vi "PythonIDE.vi"(7 "Python version":string="3.9", 9 "Processor":u16(ring) items=["SPIKE", "Pi", "Pi_ssh", "OpenMV", "duino"], 11 "Port":string) -> ()   [LabVIEW 2022 SP3]
uses:
  <vilib>/event_ctls.llb/eventvkey.ctl
  <vilib>/Utility/miscctls.llb/LVSelectionTypeDef.ctl
  06413ba0-247e-6043-8ea0-68123fbbc81b.vi
  <vilib>/Comparison/Equal/Equal Functor/Equal Functor.lvclass
  <vilib>/Platform/browser.llb/Open URL in Default Browser (string).vi
panel:
  out "live":bool
  out "last":string
  out "Text.Scroll Position":u32
  in  "Format":T1(ring)
  in  "Name":string="main.py"
  in  "Spaces":bool
  out "Shift":bool
  in  "Explorer":u16(ring) items=["Explore...", "Arm", "Backpack", "Image", "Motors", "MQTT_Client", "OnshapeTwin", "OpenMV", "Pinouts", "ROS2", "Scope", "Spatial Toolbox", "Tektronix", "Twin"]
  in  "reconnect":bool
  out "VKey":T2
  in  "Browser":bool
  out "error IO":errorcluster
  in  "Tree":string(tree)
  in  "recent":u16(ring)
  in  "CtrlE":bool
  in  "Font Size":u32=12
  in  "run":bool
  in  "Save SPIKE":bool
  out "Script":string
  in  "Python Code":string
  out "Line #":string
  out "Buffer":i32(slide) scale=0.0..100000.0
  out "History":path[](array[path])
  out "Graph":dbl[](graph)
  out "JPG":picture
  out "Chart":dbl[](graph)
  out "Console":string
  out "Path":path
  in  "Clear":bool
  in  "Ctrl C":bool
  in  "Save Log":bool
  in  "stop":bool
  # "PyVIEW IDE\nversion 0.1b37"
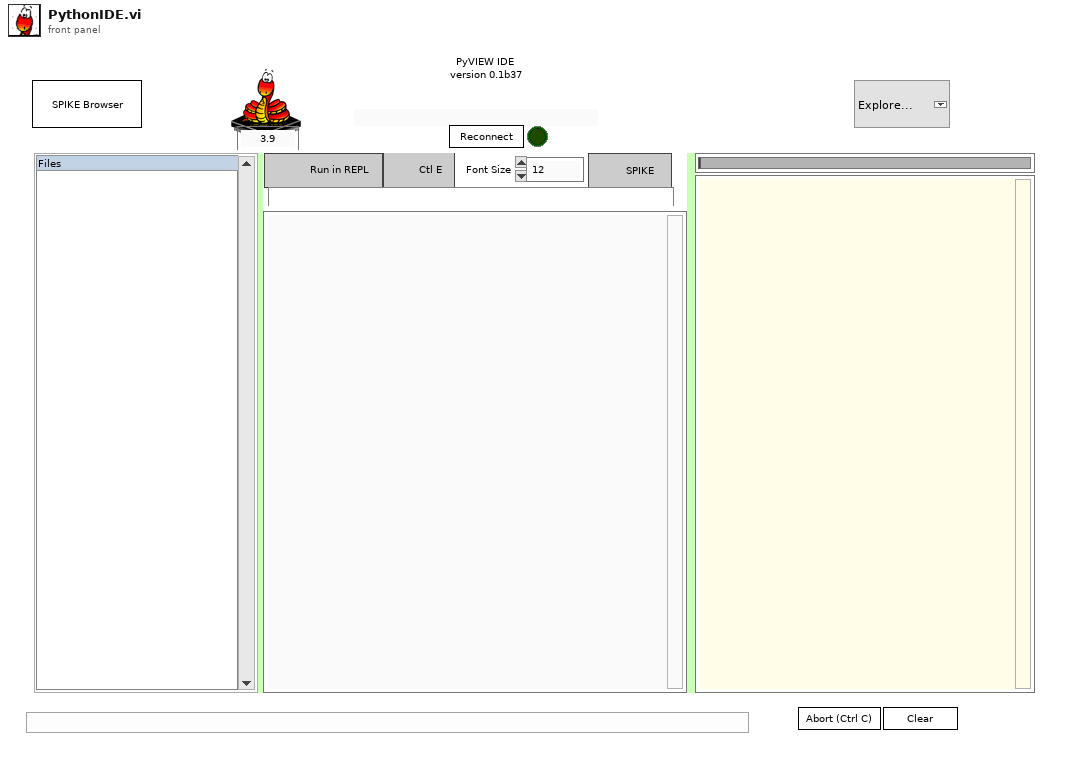
[diagram p1: front panel]
types:
  T1 = enum16{"Text", "Chart", "Waveforms", "JPEG", "Split View"}
  T2 = typedef "eventvkey.ctl" = enum16{"ASCII", "Enter", "Return", "Shift", "Ctrl", "Alt", "Cmd", "Opt", "Caps", "NumLock", "Clear", "Break", "Up", "Down", "Left", "Right", "Insert", "Delete", "Home", "End", "PageUp", "PageDown", "Escape", "Help", "Pause", "ScrollLock", "F1", "F2", "F3", "F4", "F5", "F6", "F7", "F8", "F9", "F10", "F11", "F12", "F13", "F14", "F15", "F16", "F17", "F18", "F19", "F20", "F21", "F22", "F23", "F24", "Play", "VolumeUp", "VolumeDown", "Mute", "Two Byte Char"}
  T3 = enum16{"read", "write pause", "write port", "write path", "write all"}
  T4 = typedef "PythonCtrl.ctl" = cluster{"session":refnum<k35>, "PyPath":path, "Processor":T5, "Port":string, "version":string}
  T5 = typedef "Processors.ctl" = enum16{"SPIKE", "Pi", "Pi_ssh", "OpenMV", "Dunio"}
  T6 = enum8{"Enabled", "Disabled", "Disabled and Grayed Out"}
  T7 = typedef "LVSelectionTypeDef.ctl" = cluster{"Selection Start":u32, "Selection End":u32}
  T8 = enum16{"Not data", "single values", "XY pairs", "Arrays"}
  T9 = typedef "LVPoint32TypeDef.ctl" = cluster{"Horizontal":i32, "Vertical":i32}
  T10 = typedef "Preferences.ctl" = cluster{"python":string, "arduino CLI":path, "pythonCodes":cluster{"pythonCode":path, "Color":u32}[], "FontSize":u8, "Text Colors":cluster{"Quote":u32, "function":u32, "Python":u32, "Comment":u32, "Triple Quote":u32, "Text":u32}, "SSH Logins":cluster{"IP Address":string, "Username":string, "password":string}[], "packet size":u8}
  T11 = cluster{"status":bool, "code":bool, "source":bool}
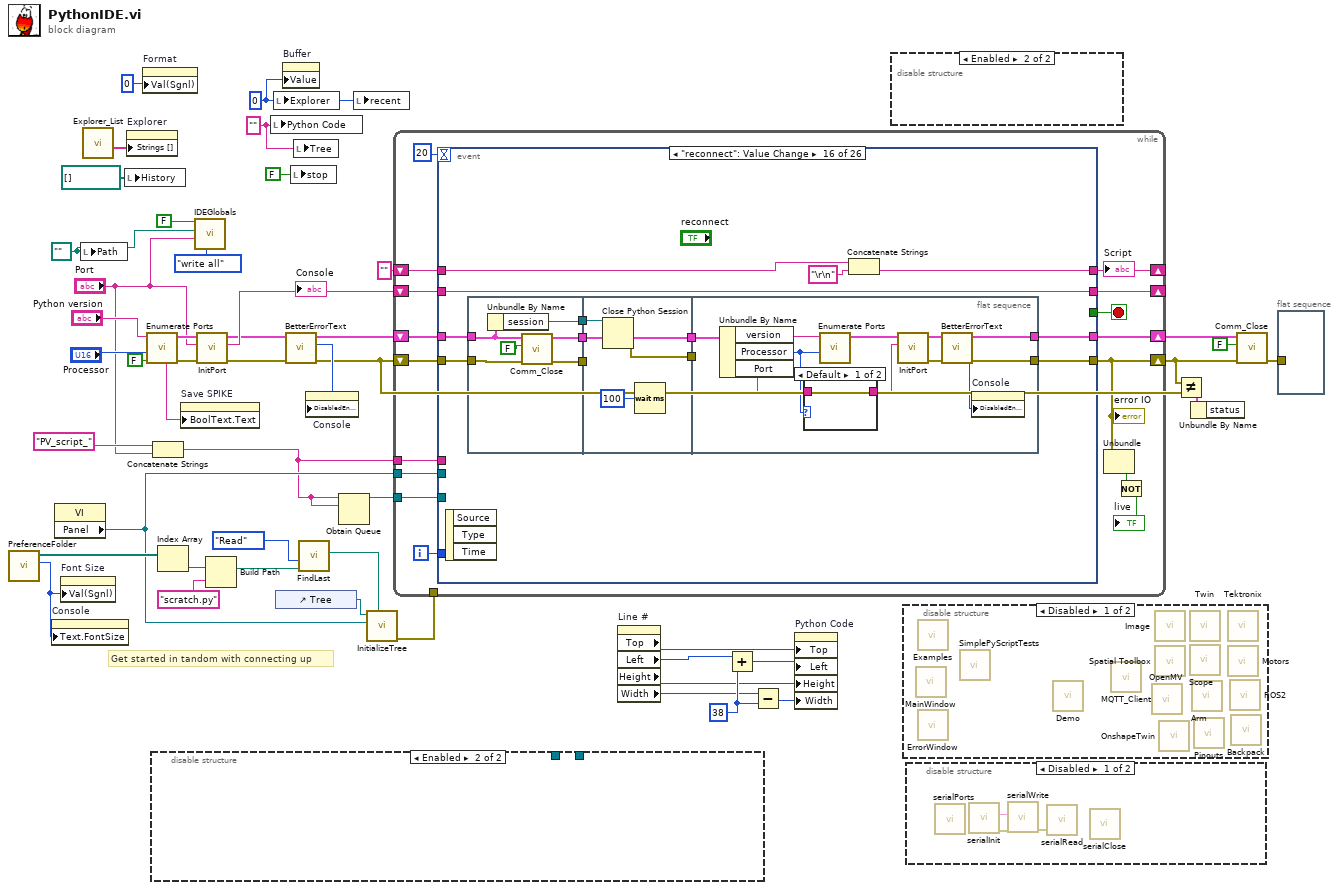
[diagram p0: block diagram]
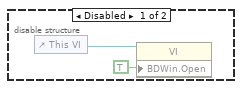
[diagram p2: hidden frame]
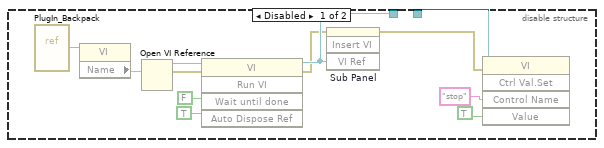
[diagram p3: hidden frame]
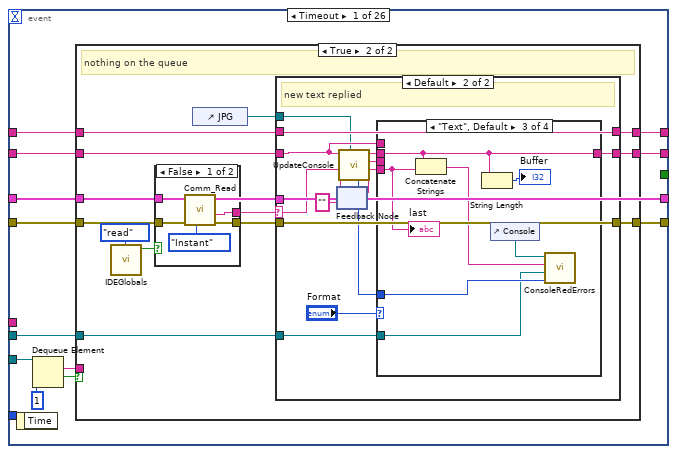
[diagram p6: hidden frame]
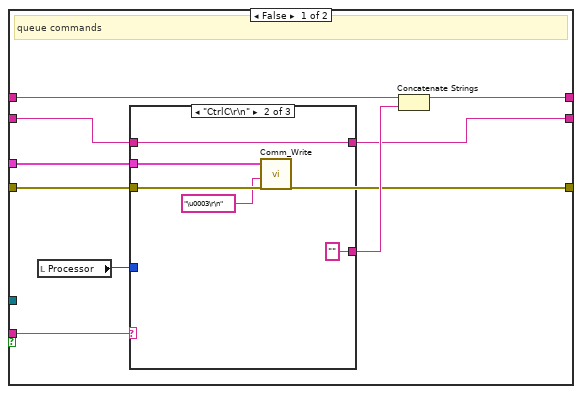
[diagram p7: hidden frame]
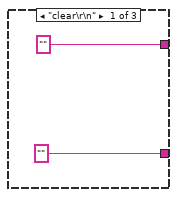
[diagram p8: hidden frame]
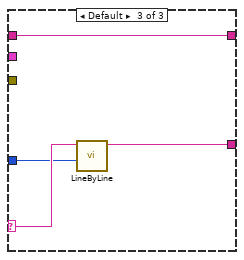
[diagram p9: hidden frame]
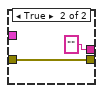
[diagram p10: hidden frame]
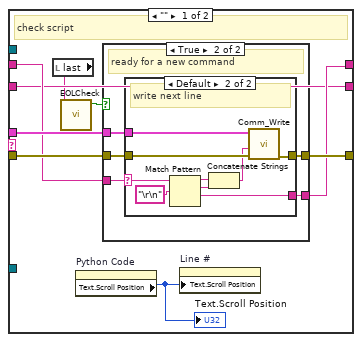
[diagram p11: hidden frame]
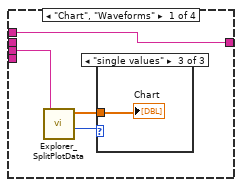
[diagram p14: hidden frame]
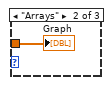
[diagram p16: hidden frame]
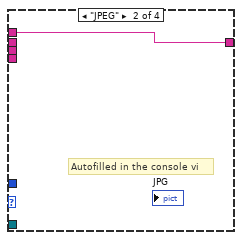
[diagram p17: hidden frame]
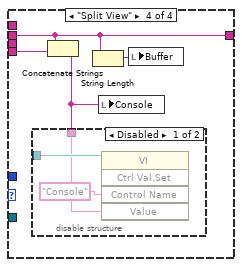
[diagram p18: hidden frame]
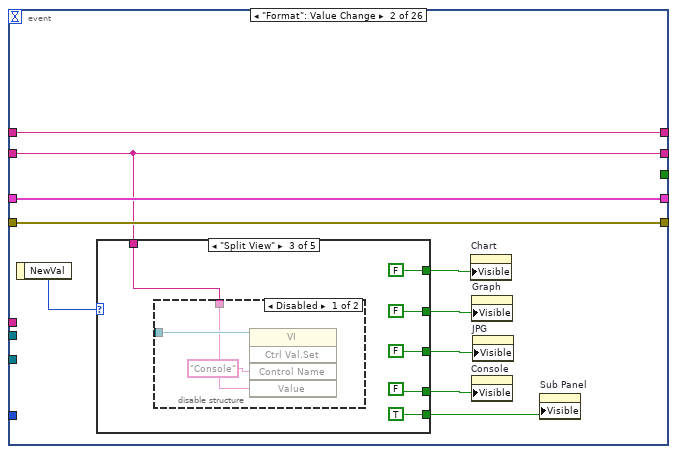
[diagram p20: hidden frame]
diagram:
  w27 = 38 ("y")
  w2 = path "" ("Path")
  w14 = 0
  w43 = "" ("Python Code")
  # "Get started in tandom with connecting up"
  n1 = call "PreferenceFolder.vi"() -> ("FontSize"=w19:u8, "pythonCodes"=w33:path[])  [unwired: 4 in, 6 out]
  n2 = property on="Console" class="Str"("Text.FontSize"=w19) -> ()  [unwired: 2 in, 2 out]
  n3 = property class="VI"() -> ("Panel"=w17:refnum<vi>)  [unwired: 2 in, 2 out]
  n4 = property on="Font Size" class="DigNum (strict)"("Val(Sgnl)"=w19) -> ()  [unwired: 2 in, 2 out]
  n5 = local write "Path"(w2) -> ()
  n6 = call "Explorer_List.vi"() -> ("Options"=w40:string[])  [unwired: 9 in, 2 out]
  n7 = local write "History"(path[] [] ("History")) -> ()
  n8 = property on="Explorer" class="Ring (strict)"("Strings []"=w40) -> ()  [unwired: 2 in, 2 out]
  n9 = property on="Format" class="Enum (strict)"("Val(Sgnl)"=0) -> ()  [unwired: 2 in, 2 out]
  n10 = call "Enumerate Ports.vi"("list?"=FALSE, "Processor"="Processor", "Python version"="Python version") -> ("error out"=w44:errorcluster, "Python"=w45:T4, "name"=w39:string)  [unwired: 3 in, 3 out]
  n11 = disable-structure shown="Enabled" {
    disable-tunnel: [w54 _] -> _
    disable-tunnel: _ -> [w51 _]
    frame Disabled {
      n12 = vi-ref "PlugIn_Backpack.vi"() -> (w55:refnum<vi>)
      n13 = property class="VI"(reference=w55) -> ("Name"=w53:string)  [unwired: 1 in, 2 out]
      n14 = Open VI Reference(vi path=w53) -> (vi reference=w57:refnum<vi>, error out=w56:errorcluster)  [unwired: 5 in]
      n15 = invoke class="VI" method="Run VI"(reference=w57, error in=w56, "Wait until done"=FALSE ("Wait Until Done"), "Auto Dispose Ref"=TRUE ("Auto Dispose Reference")) -> (reference out=w54:refnum<vi>, error out=w49:errorcluster)  [unwired: 1 in, 3 out]
      n16 = invoke on="Sub Panel" class="SubPnl" method="Insert VI"(error in=w49, "VI Ref"=w54) -> (error out=w48:errorcluster)  [unwired: 2 in, 3 out]
      n17 = invoke class="VI" method="Ctrl Val.Set"(reference=w51, error in=w48, "Control Name"="stop", "Value"=TRUE ("Auto Dispose Reference")) -> ()  [unwired: 1 in, 5 out]
    }
    frame Enabled {
    }
  }
  n18 = Concatenate Strings("PV_script_" ("name (unnamed)"), "Port") -> (w3:string)
  n19 = Index Array(array=w33) -> (element=w32:path)  [unwired: 1 in]
  n20 = property on="Save SPIKE" class="Bool"("BoolText.Text"=w39) -> ()  [unwired: 2 in, 2 out]
  n21 = call "IDEGlobals.vi"("task"=T3."write all", "Port"="Port", "Last Path"=w2, "pause?"=FALSE) -> ()  [unwired: 5 in, 3 out]
  n22 = call "InitPort.vi"("error in (no error)"=w44, "Port"="Port", "Python"=w45) -> ("error out"=w9:errorcluster, "Console"=w35:string, "Python out"=w29:T4)  [unwired: 6 in]
  "Console" <- w35
  n23 = Build Path(base path=w32, name or relative path="scratch.py" ("Python Code")) -> (appended path=w31:path)
  n24 = local write "Python Code"(w43) -> ()
  n25 = local write "Explorer"(w14) -> ()
  n26 = control-ref of="Tree"() -> (w37:refnum<vi>)
  n27 = property on="Buffer" class="Slide (strict)"("Value"=w14) -> ()  [unwired: 2 in, 2 out]
  n28 = call "BetterErrorText.vi"("error in (no error)"=w9, "Python"=w29) -> ("Disabled"=w18:T6, "Python out"=w21:T4)  [unwired: 8 in]
  n29 = local write "stop"(FALSE ("stop")) -> ()
  n30 = local write "Tree"(w43) -> ()
  n31 = call "FindLast.vi"("default"=w31, "Task"=enum16{"Save", "Read"}."Read") -> ("path"=w16:path)  [unwired: 9 in]
  n32 = property on="Console" class="Str"("DisabledEnum"=w18) -> ()  [unwired: 2 in, 2 out]
  n33 = Obtain Queue(name (unnamed)=w3, element data type=w3) -> (queue out=w41:refnum<queue>)  [unwired: 3 in, 2 out]
  n34 = local write "recent"(w14) -> ()
  n35 = call "InitializeTree.vi"("Selected File"=w16, "Panel"=w17, "TreeControl in"=w37) -> ("error out"=w11:errorcluster)  [unwired: 7 in, 1 out]
  n36 = while {
    shift-right: [w74] -> _
    shift-left: w35 -> [w75]
    shift-right: [w62] -> w10
    shift-left: w9 -> [w71]
    tunnel: w17 -> [w70]
    shift-right: [w68] -> _
    shift-left: "" -> [w69]
    tunnel: w41 -> [w66]
    shift-right: [w65] -> w13
    shift-left: w21 -> [w67]
    tunnel: w11 -> [_]
    tunnel: w3 -> [w63]
    i -> [w64]
    stop <- w73 stop-if-true
    n37 = event shown="[15] \"reconnect\": Value Change" {
      selector: _ -> [_ _ _ _ _ _ _ _ _ _ _ _ _ _ _ _ _ _ _ _ _ _ _ _ _ _]
      dyn-events: _ -> [_ _ _ _ _ _ _ _ _ _ _ _ _ _ _ _ _ _ _ _ _ _ _ _ _ _]
      timeout: 20 -> [_ _ _ _ _ _ _ _ _ _ _ _ _ _ _ _ _ _ _ _ _ _ _ _ _ _]
      tunnel: w67 -> [w77 w200 w227 w237 w253 w259 w273 w357 w366 w370 w379 w400 w417 w434 w447 w464 w496 w527 w538 w546 w553 w563 w569 w583 w592 w603]
      tunnel: w75 -> [w87 w191 w230 w244 w256 w264 w288 w360 w368 w375 w388 w398 w423 w445 w451 w465 w501 w530 w541 _ w555 w566 w578 w589 w598 w602]
      tunnel: [w86 w191 w230 w244 w256 w264 w288 w360 w368 w375 w388 w397 w423 w445 w451 w465 w501 w530 w541 w551 w555 w566 w578 w589 w598 w602] -> w74
      tunnel: [_ _ "stop" w241 _ _ _ _ _ _ _ _ _ _ _ _ _ _ _ _ _ _ _ _ _ _] -> w73
      tunnel: w71 -> [w82 w199 w229 w243 w255 w263 w282 w359 w367 w374 w387 w399 w422 w446 w452 w463 w499 w528 w539 w552 w559 w568 w580 w591 w600 w605]
      tunnel: [w85 w199 w229 w243 w255 w263 w283 w359 w367 w372 w387 w401 w422 w446 w452 w462 w499 w528 w539 w552 w559 w568 w580 w591 w600 w605] -> w62
      tunnel: w70 -> [w76 _ _ _ _ _ _ _ _ _ w386 _ _ _ _ _ _ w526 _ _ _ _ _ _ _ w608]
      tunnel: [w84 w198 w228 w242 w254 w257 w279 w361 w369 "" w385 w402 w424 w444 w450 w458 w500 w529 w540 w548 w558 w567 w579 w590 w599 w601] -> w68
      tunnel: w69 -> [w83 w198 w228 w242 w254 w262 w280 w361 w369 _ w385 w402 w424 w444 w450 w459 w500 w529 w540 w550 w558 w567 w579 w590 w599 w604]
      tunnel: w66 -> [w81 _ _ _ _ _ _ _ _ _ _ _ _ _ _ _ _ _ _ _ _ _ _ _ _ _]
      tunnel: [w77 w200 w227 w237 w253 w259 w273 w357 w366 w370 w379 w396 w417 w434 w447 w461 w496 w527 w538 w546 w553 w563 w569 w583 w592 w603] -> w65
      tunnel: w64 -> [_ _ _ _ _ _ _ _ _ _ w376 _ _ _ _ _ _ _ _ _ _ _ _ _ _ _]
      tunnel: w63 -> [_ _ _ _ _ _ _ _ _ _ _ _ w416 _ _ _ _ _ _ _ _ _ _ _ _ _]
      event Timeout {
        n38 = event-data() -> ()  [unwired: 1 in, 1 out]
        n39 = Dequeue Element(queue=w81, timeout in ms (-1)=1) -> (element=w78:string, timed out?=w79:bool)  [unwired: 1 in, 2 out]
        n40 = case shown="True" w79 {
          tunnel: w87 -> [w91 w112]
          tunnel: [w92 w114] -> w86
          tunnel: [w88 w120] -> w85
          tunnel: [w95 w119] -> w84
          tunnel: w83 -> [w96 w118]
          tunnel: w82 -> [w88 w117]
          tunnel: w77 -> [w89 w115]
          tunnel: w78 -> [w93 _]
          tunnel: w76 -> [_ w110]
          frame False {
            # "queue commands"
            n41 = local read "Processor"() -> (w90:u16)
            n42 = case shown="\"CtrlC\\r\\n\"" w93 {
              selector: w93 -> [_ _ w105]
              tunnel: ["" ("result string") "" ("result string") w107] -> w94
              tunnel: ["" ("Console") w103 w106] -> w92
              tunnel: w91 -> [_ w103 w106]
              tunnel: w90 -> [_ _ w104]
              tunnel: w89 -> [_ w100 _]
              tunnel: w88 -> [_ w99 _]
              frame "clear\r\n" {
              }
              frame "CtrlC\r\n" {
                n43 = call "Comm_Write.vi"("error in (no error)"=w99, "Text to write"="\u0003\r\n" ("function name"), "Python"=w100) -> ()  [unwired: 7 in, 2 out]
              }
              frame Default {
                n44 = call "LineByLine.vi"("Processor"=w104, "Python Code"=w105) -> ("result string"=w107:string)  [unwired: 9 in]
              }
            }
            n45 = Concatenate Strings(w96, w94) -> (w95:string)
          }
          frame True {
            # "nothing on the queue"
            n46 = call "IDEGlobals.vi"("task"=T3."read") -> ("pause? out"=w108:bool)  [unwired: 8 in, 2 out]
            n47 = case shown="False" w108 {
              tunnel: w117 -> [w125 w127]
              tunnel: [w124 "" ("Text read")] -> w113
              tunnel: [w123 w127] -> w116
              tunnel: w115 -> [w122 _]
              frame False {
                n48 = call "Comm_Read.vi"("Task"=enum16{"Instant", "All"}."Instant", "error in (no error)"=w125, "Python"=w122) -> ("error out"=w123:errorcluster, "Text read"=w124:string)  [unwired: 7 in]
              }
              frame True {
              }
            }
            n49 = control-ref of="JPG"() -> (w111:refnum<vi>)
            n50 = case shown="Default" w113 {
              selector: w113 -> [_ w162]
              tunnel: w112 -> [w130 w157]
              tunnel: w116 -> [w136 w169]
              tunnel: [w135 w169] -> w120
              tunnel: w118 -> [w133 w168]
              tunnel: [w132 w168] -> w119
              tunnel: w115 -> [w134 _]
              tunnel: [w130 w158] -> w114
              tunnel: w111 -> [_ w156]
              tunnel: w110 -> [_ w155]
              frame "" {
                # "check script"
                n51 = local read "last"() -> (w128:string)
                n52 = call "EOLCheck.vi"("Console"=w128) -> ("waiting...."=w129:bool)  [unwired: 10 in]
                n53 = property on="Python Code" class="Str"() -> ("Text.Scroll Position"=w131:u32)  [unwired: 2 in, 2 out]
                "Text.Scroll Position" <- w131
                n54 = case shown="True" w129 {
                  tunnel: w136 -> [w138 w143]
                  tunnel: [w138 w142] -> w135
                  tunnel: w134 -> [_ w141]
                  tunnel: w133 -> [w137 w140]
                  tunnel: [w137 w139] -> w132
                  frame False {
                  }
                  frame True {
                    # "ready for a new command"
                    n55 = case shown="Default" w140 {
                      selector: w140 -> [w144 w146]
                      tunnel: [w144 w154] -> w139
                      tunnel: w143 -> [w145 w150]
                      tunnel: [w145 w149] -> w142
                      tunnel: w141 -> [_ w147]
                      frame "" {
                      }
                      frame Default {
                        # "write next line"
                        n56 = Match Pattern(string=w146, regular expression="\r\n") -> (before substring=w152:string, match substring=w151:string, after substring=w154:string)  [unwired: 1 in, 1 out]
                        n57 = Concatenate Strings(w152, w151) -> (w148:string)
                        n58 = call "Comm_Write.vi"("error in (no error)"=w150, "Text to write"=w148, "Python"=w147) -> ("error out"=w149:errorcluster)  [unwired: 7 in, 1 out]
                      }
                    }
                  }
                }
                n59 = property on="Line #" class="Str"("Text.Scroll Position"=w131) -> ()  [unwired: 2 in, 2 out]
              }
              frame Default {
                # "new text replied"
                n60 = feedback #1("" ("Left over raw")) -> (w166:string)
                n61 = call "UpdateConsole.vi"("JPG"=w156, "from last time raw"=w166, "New Text"=w162, "Console"=w157) -> ("Left over raw"=w167:string, "left over fixed"=w160:string, "LastFullLine"=w161:string, "Console Out"=w159:string, "cursor out"=w164:i32)  [unwired: 2 in, 1 out]
                n62 = feedback-in #1(w167) -> ()
                n63 = case shown="\"Text\", Default" "Format" {
                  tunnel: w164 -> [_ _ w183 _]
                  tunnel: w161 -> [w173 _ _ _]
                  tunnel: w159 -> [_ _ w180 w186]
                  tunnel: w160 -> [_ _ w181 w187]
                  tunnel: [w170 w176 w180 w186] -> w158
                  tunnel: w157 -> [w170 w176 _ _]
                  tunnel: w155 -> [_ _ w178 _]
                  frame "Chart", "Waveforms" {
                    n64 = call "Explorer_SplitPlotData.vi"("Value"=w173) -> ("Data type"=w171:T8, "Array"=w172:dbl[])  [unwired: 9 in]
                    n65 = case shown="\"single values\"" w171 {
                      tunnel: w172 -> [_ w174 w175]
                      frame Default {
                      }
                      frame "Arrays" {
                        "Graph" <- w174
                      }
                      frame "single values" {
                        "Chart" <- w175
                      }
                    }
                  }
                  frame "JPEG" {
                    # "Autofilled in the console vi"
                  }
                  frame "Text", Default {
                    n66 = Concatenate Strings(w180, w181) -> (w177:string)
                    n67 = String Length(string=w180) -> (length=→"Buffer":i32)
                    n68 = control-ref of="Console"() -> (w179:refnum<vi>)
                    n69 = call "ConsoleRedErrors.vi"("Text.Selection:End"=w183, "Front Panel"=w178, "Console in"=w177, "String in"=w179) -> ()  [unwired: 6 in, 2 out]
                    "last" <- w181
                  }
                  frame "Split View" {
                    n70 = Concatenate Strings(w186, w187) -> (w184:string)
                    n71 = disable-structure shown="Disabled" {
                      disable-tunnel: _ -> [w189 _]
                      disable-tunnel: w184 -> [w188 _]
                      frame Disabled {
                        n72 = invoke class="VI" method="Ctrl Val.Set"(reference=w189, "Control Name"="Console", "Value"=w188) -> ()  [unwired: 2 in, 5 out]
                      }
                      frame Enabled {
                      }
                    }
                    n73 = String Length(string=w186) -> (length=w185:i32)
                    n74 = local write "Console"(w184) -> ()
                    n75 = local write "Buffer"(w185) -> ()
                  }
                }
              }
            }
          }
        }
      }
      event "Format": Value Change {
        n76 = event-data() -> ("NewVal"=w197:T1)  [unwired: 1 in]
        n77 = case shown="\"Split View\"" w197 {
          tunnel: [TRUE ("Visible") FALSE ("Visible") FALSE ("Visible") FALSE ("Visible") FALSE ("Visible")] -> w196
          tunnel: [FALSE ("Visible") TRUE ("Visible") FALSE ("Visible") FALSE ("Visible") FALSE ("Visible")] -> w195
          tunnel: [FALSE ("Visible") FALSE ("Visible") FALSE ("Visible") TRUE ("Visible") FALSE ("Visible")] -> w194
          tunnel: [FALSE ("Visible") FALSE ("Visible") FALSE ("Visible") FALSE ("Visible") TRUE ("Visible")] -> w193
          tunnel: [_ FALSE ("Visible") TRUE ("Visible") _ _] -> w192
          tunnel: w191 -> [_ _ w210 _ _]
          frame "JPEG" {
          }
          frame "Waveforms" {
          }
          frame "Split View" {
            n78 = disable-structure shown="Disabled" {
              disable-tunnel: _ -> [w217 _]
              disable-tunnel: w210 -> [w216 _]
              frame Disabled {
                n79 = invoke class="VI" method="Ctrl Val.Set"(reference=w217, "Control Name"="Console", "Value"=w216) -> ()  [unwired: 2 in, 5 out]
              }
              frame Enabled {
              }
            }
          }
          frame "Chart" {
          }
          frame "Text" {
          }
        }
        n80 = property on="Chart" class="WFChart (strict)"("Visible"=w194) -> ()  [unwired: 2 in, 2 out]
        n81 = property on="Graph" class="WFGraph (strict)"("Visible"=w195) -> ()  [unwired: 2 in, 2 out]
        n82 = property on="Console" class="Str"("Visible"=w193) -> ()  [unwired: 2 in, 2 out]
        n83 = property on="JPG" class="Pict"("Visible"=w196) -> ()  [unwired: 2 in, 2 out]
        n84 = property on="Sub Panel" class="SubPnl"("Visible"=w192) -> ()  [unwired: 2 in, 2 out]
      }
      event "stop": Value Change {
        n85 = event-data() -> ()  [unwired: 1 in, 1 out]
      }
      event Panel Close? {
        w236 = "" ("source")
        w241 = TRUE ("stop")
        n86 = event-data() -> ()  [unwired: 1 in, 3 out]
        n87 = control-ref of="Tree"() -> (w240:refnum<vi>)
        n88 = property on="recent" class="Ring (strict)"("Strings []"=string[] []) -> ()  [unwired: 2 in, 2 out]
        n89 = invoke on="Invoke Node" class="Tree (strict)" method="Edit Tree Items.Delete"(reference=w240, "Delete Children"=TRUE ("Delete Children?")) -> ()  [unwired: 3 in, 5 out]
        n90 = local write "Python Code"(w236) -> ()
        n91 = local write "Console"(w236) -> ()
        n92 = local write "Path"(path "") -> ()
        n93 = local write "Line #"(w236) -> ()
        n94 = local write "History"(path[] [] ("History")) -> ()
        n95 = property on="Console" class="Str"("Visible"=TRUE ("Delete Children?")) -> ()  [unwired: 2 in, 2 out]
        n96 = property on="Sub Panel" class="SubPnl"("Visible"=FALSE ("Delete Children?")) -> ()  [unwired: 2 in, 2 out]
        n97 = event-data("Discard?"=w241) -> ()  [unwired: 1 in, 1 out]
      }
      event Pane Size; Panel Resize {
        w247 = 38 ("y")
        n98 = event-data() -> ()  [unwired: 1 in, 5 out]
        n99 = property on="Line #" class="Str"() -> ("Top"=w250:i32, "Left"=w252:i32, "Height"=w249:u32, "Width"=w248:u32)  [unwired: 2 in, 2 out]
        n100 = local read "Text.Scroll Position"() -> (w245:u32)
        n101 = Add(x=w252, y=w247) -> (x+y=w251:i32)
        n102 = Subtract(x=w248, y=w247) -> (x-y=w246:u32)
        n103 = property on="Python Code" class="Str"("Text.Scroll Position"=w245, "Top"=w250, "Left"=w251, "Height"=w249, "Width"=w246) -> ()  [unwired: 2 in, 2 out]
      }
      event "run": Value Change {
        n104 = event-data() -> ()  [unwired: 1 in, 1 out]
        n105 = local read "Processor"() -> (w260:u16)
        n106 = case shown="False" "CtrlE" {
          tunnel: [w267 w270] -> w257
          tunnel: "Python Code" -> [w266 w271]
          tunnel: w260 -> [w265 _]
          frame False {
            n107 = call "LineByLine.vi"("Processor"=w265, "Python Code"=w266) -> ("result string"=w267:string)  [unwired: 9 in]
          }
          frame True {
            n108 = Concatenate Strings("\u0005" ("string"), w271, "\u0004" ("string")) -> (w270:string)
          }
        }
        n109 = Concatenate Strings(w262, w257) -> ()  [unwired: 1 out]
      }
      event Key Down? {
        n110 = event-data() -> ("PlatMods.Shift"=w274:bool, "PlatMods.Cmd"=w284:bool, "PlatMods.Ctrl"=w285:bool, "Char"=w286:i16, "VKey"=w287:T2)  [unwired: 1 in]
        "VKey" <- w287
        "Shift" <- w274
        n111 = property on="Python Code" class="Str"() -> ("Key Focus"=w276:bool)  [unwired: 2 in, 2 out]
        n112 = property on="Sub Panel" class="SubPnl"() -> ("Key Focus"=w272:bool)  [unwired: 2 in, 2 out]
        n113 = property on="Name" class="Str"() -> ("Key Focus"=w277:bool)  [unwired: 2 in, 2 out]
        n114 = Compound Arithmetic op=OR(w272, w276, w277) -> (w275:bool)
        n115 = case shown="True" w275 {
          tunnel: w273 -> [w297 _]
          tunnel: w287 -> [w299 _]
          tunnel: w286 -> [w298 w350]
          tunnel: w285 -> [w290 _]
          tunnel: w284 -> [w291 _]
          tunnel: [w295 w352] -> w283
          tunnel: w282 -> [w296 w352]
          tunnel: [w292 w349] -> w281
          tunnel: w280 -> [w294 w351]
          tunnel: [w293 w351] -> w279
          tunnel: w274 -> [_ w348]
          frame False {
            n116 = Or(x=w291, y=w290) -> (x .or. y?=w289:bool)
            n117 = case shown="True" w289 {
              tunnel: w299 -> [w306 _]
              tunnel: w298 -> [w305 w322]
              tunnel: w297 -> [w304 w321]
              tunnel: w296 -> [w303 w320]
              tunnel: [w301 w319] -> w295
              tunnel: w294 -> [w300 w318]
              tunnel: [w300 w317] -> w293
              tunnel: w291 -> [_ w316]
              tunnel: [_ w315] -> w292
              frame False {
                n118 = case shown="\"Left\"" w306 {
                  tunnel: w305 -> [_ _ _ _ _ w314]
                  tunnel: ["\r\n" ("replace string (\"\")") "\u001b[A" ("replace string (\"\")") "\u001b[B" ("replace string (\"\")") "\u001b[D" ("replace string (\"\")") "\u001b[C" ("replace string (\"\")") w312] -> w302
                  frame "Enter", "Return" {
                  }
                  frame "Up" {
                  }
                  frame "Down" {
                  }
                  frame "Left" {
                  }
                  frame "Right" {
                  }
                  frame Default {
                    n119 = Build Array(w314) -> (w313:i16[])
                    n120 = Byte Array To String(unsigned byte array=w313) -> (string=w312:string)
                  }
                }
                n121 = call "Comm_Write.vi"("error in (no error)"=w303, "Text to write"=w302, "Python"=w304) -> ("error out"=w301:errorcluster)  [unwired: 7 in, 1 out]
              }
              frame True {
                n122 = case shown="Default" w322 {
                  selector: w322 -> [w325 _]
                  tunnel: w321 -> [w330 _]
                  tunnel: w320 -> [w329 w347]
                  tunnel: [w328 w347] -> w319
                  tunnel: w318 -> [w326 w346]
                  tunnel: [w326 w345] -> w317
                  tunnel: w316 -> [w324 _]
                  tunnel: [w323 _] -> w315
                  frame Default {
                    n123 = case shown="False" w324 {
                      tunnel: [w332 "" ("string")] -> w327
                      tunnel: w325 -> [w331 _]
                      tunnel: [_ TRUE ("Discard?")] -> w323
                      frame False {
                        # "Ctrl - clean up"
                        n124 = case shown="98" w331 {
                          tunnel: w331 -> [_ _ _ _ w338]
                          tunnel: ["\u0003" ("string") "\u0002" ("string") "\u0004" ("string") "\u0005" ("string") w337] -> w332
                          frame 67, 99 {
                          }
                          frame 98 {
                            # "Ctrl B PC"
                          }
                          frame 68, 100 {
                          }
                          frame 101 {
                            # "Ctrl E PC"
                          }
                          frame Default {
                            # "Ctrl C PC"
                            n125 = Build Array(w338) -> (w339:i16[])
                            n126 = Byte Array To String(unsigned byte array=w339) -> (string=w337:string)
                          }
                        }
                      }
                      frame True {
                        # "Cmd C/V use OS"
                      }
                    }
                    n127 = call "Comm_Write.vi"("error in (no error)"=w329, "Text to write"=w327, "Python"=w330) -> ("error out"=w328:errorcluster)  [unwired: 7 in, 1 out]
                  }
                  frame 22, 118 {
                    # "paste"
                    n128 = invoke class="App" method="Clipboard.Read"() -> ("Read Clipbrd"=w344:string)  [unwired: 3 in, 2 out]
                    n129 = local read "Processor"() -> (w342:u16)
                    n130 = call "LineByLine.vi"("Processor"=w342, "Python Code"=w344) -> ("result string"=w343:string)  [unwired: 9 in]
                    n131 = Concatenate Strings(w346, w343) -> (w345:string)
                  }
                }
              }
            }
          }
          frame True {
            n132 = case shown="9" w350 {
              tunnel: [TRUE ("Discard?") _] -> w349
              tunnel: w348 -> [_ w355]
              frame 0, Default {
              }
              frame 9 {
                # "Tab key"
                n133 = control-ref of="Python Code"() -> (w356:refnum<vi>)
                n134 = call "Tab_In_Out.vi"("Shift?"=w355, "String in"=w356) -> ("result string"=w354:string)  [unwired: 9 in]
                n135 = property on="Python Code" class="Str"("Val(Sgnl)"=w354) -> ()  [unwired: 2 in, 2 out]
              }
            }
          }
        }
        n136 = Not(x=w281) -> (.not. x?=w278:bool)
        n137 = event-data("Discard?"=w278) -> ()  [unwired: 1 in, 1 out]
      }
      event Key Up {
        n138 = event-data() -> ()  [unwired: 1 in, 8 out]
        n139 = local write "Shift"(FALSE ("Shift")) -> ()
      }
      event "recent": Value Change {
        n140 = event-data() -> ()  [unwired: 1 in, 6 out]
        n141 = local read "History"() -> (w364:path[])
        n142 = Index Array(array=w364, index="recent") -> (element=w363:path)
        n143 = Path To String(path=w363) -> (string=w362:string)
        n144 = property on="Tree" class="Tree (strict)"("Val(Sgnl)"=w362) -> ()  [unwired: 2 in, 2 out]
      }
      event "Ctrl C": Value Change {
        n145 = event-data() -> ()  [unwired: 1 in, 1 out]
        n146 = call "Comm_Write.vi"("error in (no error)"=w374, "Text to write"="\u0003\r\n\r\n" ("function name"), "Python"=w370) -> ("error out"=w372:errorcluster)  [unwired: 7 in, 1 out]
      }
      event "Python Code": Value Change {
        n147 = event-data() -> ()  [unwired: 1 in, 1 out]
        n148 = local read "VKey"() -> (w383:T2)
        n149 = case shown="\"Enter\", \"Return\"" w383 {
          tunnel: [FALSE TRUE] -> w382
          frame Default {
          }
          frame "Enter", "Return" {
          }
        }
        n150 = control-ref of="Python Code"() -> (w384:refnum<vi>)
        n151 = call "Color_Assign.vi"("Add Spaces?"=w382, "Front Panel"=w386, "Code"=w384) -> ("Value"=w378:string)  [unwired: 8 in]
        n152 = call "BuildLineNumbers.vi"("Python Code"=w378) -> ("String"=→"Line #":string)  [unwired: 10 in]
        n153 = property on="Python Code" class="Str"() -> ("DisabledEnum"=w380:T6)  [unwired: 2 in, 2 out]
        n154 = local read "Tree"() -> (w381:string)
        n155 = case shown="\"Enabled\"" w380 {
          tunnel: w378 -> [_ w392]
          tunnel: w381 -> [_ w391]
          tunnel: w376 -> [_ w389]
          frame Default {
          }
          frame "Enabled" {
            n156 = case shown="0..5" w389 {
              frame Default {
              }
              frame 0..5 {
                n157 = property on="Ctrl C" class="Bool"("Key Focus"=TRUE) -> ()  [unwired: 2 in, 2 out]
              }
            }
            n158 = String To Path(string=w391) -> (path=w390:path)
            n159 = Write to Text File(file (use dialog)=w390, text=w392) -> ()  [unwired: 2 in, 3 out]
          }
        }
      }
      event "Save SPIKE": Value Change {
        n160 = event-data() -> ()  [unwired: 1 in, 3 out]
        n161 = case shown="No Error" w399 {
          selector: w399 -> [w410 w415]
          tunnel: [w412 w415] -> w401
          tunnel: w398 -> [_ w414]
          tunnel: w400 -> [w411 w413]
          tunnel: [w404 w414] -> w397
          tunnel: [w403 w413] -> w396
          frame No Error {
            n162 = local read "Tree"() -> (w407:string)
            n163 = local read "Python Code"() -> (w409:string)
            n164 = String To Path(string=w407) -> (path=w408:path)
            n165 = Strip Path(path=w408) -> (name=w406:string)  [unwired: 1 out]
            n166 = control-ref of="Console"() -> (w405:refnum<vi>)
            n167 = call "UploadFiles.vi"("Code"=w409, "error in (no error)"=w410, "Python in"=w411, "name"=w406, "Console"=w405) -> ("error out"=w412:errorcluster, "Console out"=w404:string, "Python out"=w403:T4)  [unwired: 4 in]
          }
          frame Error {
          }
        }
      }
      event "Explorer": Value Change {
        n168 = event-data() -> ("NewVal"=w419:u16)  [unwired: 1 in]
        n169 = property on="Explorer" class="Ring (strict)"() -> ("Strings []"=w420:string[])  [unwired: 2 in, 2 out]
        n170 = Index Array(array=w420, index=w419) -> (element=w418:string)
        n171 = case shown="Default" w419 {
          tunnel: w418 -> [_ w431]
          tunnel: w416 -> [_ w425]
          frame 0 {
          }
          frame Default {
            n172 = local read "Shift"() -> (w430:bool)
            n173 = Select(t=enum16{"run", "open"}."open" ("Task"), s=w430, f=enum16{"run", "open"}."run" ("Task")) -> (s? t:f=w427:enum16{"run", "open"})
            n174 = control-ref of="Console"() -> (w432:refnum<vi>)
            n175 = control-ref of="JPG"() -> (w426:refnum<vi>)
            n176 = call "Explore_Open.vi"("JPG"=w426, "Task"=w427, "queueName"=w425, "Name"=w431, "String in"=w432) -> ()  [unwired: 7 in]
          }
        }
        n177 = local write "Explorer"(0) -> ()
      }
      event "Browser": Value Change {
        w442 = 128  # call and forget
        n178 = event-data() -> ()  [unwired: 1 in, 3 out]
        n179 = vi-ref "Examples.vi"() -> (w439:refnum<vi>)
        n180 = property class="VI"(reference=w439) -> ("Name"=w440:string)  [unwired: 1 in, 2 out]
        n181 = local read "Python version"() -> (w433:string)
        n182 = local read "Port"() -> (w438:string)
        n183 = Open VI Reference(type specifier VI Refnum (for type only)=refnum<vi> refnum, vi path=w440, options=w442) -> (vi reference=w443:refnum<vi>, error out=w435:errorcluster)  [unwired: 3 in]
        n184 = call-by-ref "Start Asynchronous Call"(reference=w443, error in=w435, "Python version"=w433, "Python"=w434, "Port"=w438) -> (reference out=w436:refnum<vi>, error out=w437:errorcluster)  [unwired: 9 in]
        n185 = Close Reference(reference=w436, error in (no error)=w437) -> ()  [unwired: 1 out]
      }
      event "Spaces": Value Change {
        n186 = event-data() -> ()  [unwired: 1 in, 3 out]
        n187 = property on="Python Code" class="Str"() -> ("Value"=w448:string)  [unwired: 2 in, 2 out]
        n188 = call "CleanUp.vi"("Python Code"=w448) -> ("spreadsheet string"=w449:string)  [unwired: 10 in]
        n189 = property on="Python Code" class="Str"("Val(Sgnl)"=w449) -> ()  [unwired: 2 in, 2 out]
      }
      event "reconnect": Value Change {
        n190 = event-data() -> ()  [unwired: 1 in, 3 out]
        n191 = flat-sequence {
          tunnel: w464 -> [w468]
          tunnel: w463 -> [w470]
          tunnel: [w469] -> w457
          tunnel: [w468] -> w455
          tunnel: [w467] -> w453
          tunnel: w457 -> [w473]
          tunnel: [w472] -> w456
          tunnel: w455 -> [w472]
          tunnel: [w471] -> w454
          tunnel: w453 -> [_]
          tunnel: [w482] -> w462
          tunnel: [w481] -> w461
          tunnel: w456 -> [w479]
          tunnel: w454 -> [_]
          frame #0 {
            n192 = Unbundle By Name(w468) -> ("session"=w469:refnum<k35>)
            n193 = call "Comm_Close.vi"("error in (no error)"=w470, "Show Err?"=FALSE, "Python in"=w468) -> ("error out"=w467:errorcluster)  [unwired: 7 in, 1 out]
          }
          frame #1 {
            n194 = Close Python Session(session in=w473) -> (11:w471:errorcluster)  [unwired: 1 in]
            n195 = Wait (ms)(milliseconds to wait=u32 100) -> ()  [unwired: 1 out]
          }
          frame #2 {
            n196 = Unbundle By Name(w479) -> ("version"=w478:string, "Processor"=w475:T5, "Port"=w477:string)
            n197 = case shown="Default" w475 {
              tunnel: w477 -> [w485 w487]
              tunnel: [w485 w486] -> w476
              frame Default {
              }
              frame "Pi_ssh" {
                n198 = call "CheckIP.vi"("port"=w487) -> ("port out"=w486:string)  [unwired: 10 in]
              }
            }
            n199 = call "Enumerate Ports.vi"("Processor"=w475, "Python version"=w478) -> ("Python"=w484:T4)  [unwired: 4 in, 5 out]
            n200 = call "InitPort.vi"("Port"=w476, "Python"=w484) -> ("error out"=w482:errorcluster, "Python out"=w483:T4)  [unwired: 7 in, 1 out]
            n201 = call "BetterErrorText.vi"("error in (no error)"=w482, "Python"=w483) -> ("Disabled"=w480:T6, "Python out"=w481:T4)  [unwired: 8 in]
            n202 = property on="Console" class="Str"("DisabledEnum"=w480) -> ()  [unwired: 2 in, 2 out]
          }
        }
        n203 = Concatenate Strings(w459, "\r\n" ("string")) -> (w458:string)
      }
      event "Tree": Value Change {
        # "need this to keep\nfrom adding spaces"
        # "rebuild tree and load new file"
        n204 = event-data() -> ()  [unwired: 1 in, 1 out]
        n205 = local read "History"() -> (w491:path[])
        n206 = String To Path(string="Tree") -> (path=w488:path)
        "Path" <- w488
        n207 = call "Search Unsorted 1D Array.vim"("element"=w488, "unsorted 1D array"=w491) -> ("index of element"=w490:i32)  [unwired: 9 in]
        n208 = local write "VKey"(eventvkey."ASCII" ("VKey")) -> ()
        n209 = case shown="Default" w490 {
          selector: w490 -> [w502 _]
          tunnel: w491 -> [_ w506]
          tunnel: w488 -> [_ w505]
          frame Default {
            n210 = property on="recent" class="Ring (strict)"("Value"=w502) -> ()  [unwired: 2 in, 2 out]
          }
          frame -1 {
            n211 = Build Array (concatenate)(w505, w506) -> (w504:path[])
            "History" <- w504
            n212 = for {
              tunnel: w504 -> [w508] mode=indexing
              tunnel: [w507] -> w503 mode=indexing
              n213 = Strip Path(path=w508) -> (name=w507:string)  [unwired: 1 out]
            }
            n214 = property on="recent" class="Ring (strict)"("Strings []"=w503) -> ()  [unwired: 2 in, 2 out]
          }
        }
        n215 = call "IDEGlobals.vi"("task"=T3."write path", "Last Path"=w488) -> ()  [unwired: 7 in, 3 out]
        n216 = Read from Text File(file (use dialog)=w488) -> (text=w498:string, error out=w497:errorcluster)  [unwired: 3 in, 2 out]
        n217 = case shown="No Error" w497 {
          tunnel: w498 -> [w519 _]
          tunnel: "Tree" -> [w517 _]
          tunnel: [TRUE ("enabled") FALSE ("enabled")] -> w493
          frame No Error {
            n218 = call "FindLast.vi"("Task"=enum16{"Save", "Read"}."Save", "Tree"=w517) -> ()  [unwired: 9 in, 1 out]
            n219 = property on="Python Code" class="Str"("Val(Sgnl)"=w519, "DisabledEnum"=T6."Enabled" ("Disabled"), "Text.Selection"=T7 {"Selection Start"=0, "Selection End"=0}, "Text.Scroll Position"=u32 0, "Key Focus"=FALSE) -> ()  [unwired: 2 in, 2 out]
          }
          frame Error {
            n220 = property on="Python Code" class="Str"("Val(Sgnl)"="" ("Python Code"), "DisabledEnum"=T6."Disabled and Grayed Out" ("Disabled")) -> ()  [unwired: 2 in, 2 out]
          }
        }
        n221 = for {
          tunnel: w493 -> [w510]
          tunnel: string[] ["WINDOW", "OPEN", "RENAME", "DUPLICATE", "DELETE_TREE", "SAVEAS_TREE", "SPACES", "RUN"] -> [w509] mode=indexing
          n222 = Current VI's Menubar() -> (w511:refnum<k9>)
          n223 = Set Menu Item Info(7:w509, 9:w510, 11:w511) -> ()  [unwired: 4 in, 2 out]
        }
      }
      event "Tree": Double Click {
        # "rebuild tree and load new file"
        n224 = event-data() -> ()  [unwired: 1 in, 1 out]
        n225 = local read "Tree"() -> (w524:string)
        n226 = String To Path(string=w524) -> (path=w525:path)
        n227 = Read from Text File(file (use dialog)=w525) -> (error out=w523:errorcluster)  [unwired: 3 in, 3 out]
        n228 = case shown="No Error" w523 {
          tunnel: w526 -> [w532 _]
          tunnel: w524 -> [w531 _]
          frame No Error {
            n229 = control-ref of="Tree"() -> (w533:refnum<vi>)
            n230 = call "Tree_Rename.vi"("Tree in"=w531, "Panel"=w532, "TreeControl in"=w533) -> ()  [unwired: 9 in]
          }
          frame Error {
          }
        }
      }
      event "Tree": Drop {
        # "Dragging"
        n231 = event-data() -> ("Coords"=w536:T9)  [unwired: 1 in]
        n232 = invoke on="Tree" class="Tree (strict)" method="Point To Row Column"("Point"=w536) -> ("InBounds"=w534:bool, "Tag"=w535:string)  [unwired: 7 in, 6 out]
        n233 = case shown="True" w534 {
          tunnel: w535 -> [_ w543]
          frame False {
          }
          frame True {
            # "original path"
            # "tag where released"
            n234 = local read "Tree"() -> (w542:string)
            n235 = flat-sequence {
              tunnel: w542 -> [_]
              tunnel: w543 -> [_]
              frame #0 {
              }
            }
          }
        }
        n236 = event-data("Accepted?"=FALSE) -> ()  [unwired: 1 in, 1 out]
      }
      event "Clear": Value Change {
        w551 = ""
        n237 = event-data() -> ()  [unwired: 1 in, 3 out]
        n238 = Concatenate Strings(w550, "\r\n" ("string")) -> (w548:string)
        n239 = local write "Graph"(dbl[] [] ("Graph")) -> ()
        n240 = property on="Chart" class="WFChart (strict)"("History Data"=dbl[] []) -> ()  [unwired: 2 in, 2 out]
        n241 = local write "Console"(w551) -> ()
        n242 = local write "Buffer"(0) -> ()
      }
      event "Save Log": Value Change {
        n243 = event-data() -> ()  [unwired: 1 in, 3 out]
        n244 = call "File Dialog3"("default name"="log.txt") -> ("selected path"=w554:path, "error out"=w556:errorcluster)  [unwired: 11 in, 2 out]
        n245 = case shown="No Error" w556 {
          tunnel: w555 -> [w561 _]
          tunnel: w554 -> [w560 _]
          frame No Error {
            n246 = Write to Text File(file (use dialog)=w560, text=w561) -> ()  [unwired: 2 in, 3 out]
          }
          frame Error {
          }
        }
      }
      event "Font Size": Value Change {
        n247 = event-data() -> ()  [unwired: 1 in, 3 out]
        n248 = call "Preferences.vi"() -> ("Preferences out"=w564:T10)  [unwired: 10 in, 1 out]
        n249 = Bundle By Name(cluster=w564, "FontSize"="Font Size") -> (w565:T10)
        n250 = property on="Python Code" class="Str"("Text.FontSize"="Font Size") -> ()  [unwired: 2 in, 2 out]
        n251 = call "Preferences.vi"("Preferences in"=w565) -> ()  [unwired: 9 in, 2 out]
        n252 = property on="Console" class="Str"("Text.FontSize"="Font Size") -> ()  [unwired: 2 in, 2 out]
      }
      event "Tree": Shortcut Menu Activation? {
        n253 = event-data() -> ("MenuRef"=w574:refnum<k9>)  [unwired: 1 in]
        n254 = local read "Tree"() -> (w572:string)
        n255 = String To Path(string=w572) -> (path=w571:path)
        n256 = call <vilib>:"Get File Extension.vi"("file"=w571) -> ("lowercase file extension"=w570:string)  [unwired: 6 in, 4 out]
        n257 = case shown="\"py\"" w570 {
          tunnel: [string[] ["Search...", "Open in Finder"] ("L10n_Parent Menus") string[] ["Search...", "Open in Finder", "Open in new window", "Duplicate", "Rename...", "Save As...", "Delete", "New..."] ("L10n_Parent Menus")] -> w573
          frame Default {
          }
          frame "py" {
          }
        }
        n258 = Delete Menu Items(9:w574) -> (0:w577:errorcluster, 3:w576:refnum<k9>)  [unwired: 3 in]
        n259 = Insert Menu Items(6:w577, 7:string[] ["SEARCH", "OPEN", "WINDOW", "DUPLICATE", "RENAME", "SAVEAS_TREE", "DELETE_TREE", "NEW_TREE"], 8:w573, 9:w576) -> ()  [unwired: 2 in, 3 out]
        n260 = event-data() -> ()  [unwired: 2 in, 1 out]
      }
      event "Console": Shortcut Menu Activation? {
        n261 = event-data() -> ("MenuRef"=w585:refnum<k9>)  [unwired: 1 in]
        n262 = Delete Menu Items(9:w585) -> (0:w588:errorcluster, 3:w587:refnum<k9>)  [unwired: 3 in]
        n263 = Insert Menu Items(6:w588, 7:string[] ["CTRLC", "CLEAR", "SAVEAS", "ERROR"], 8:string[] ["Ctrl C", "Clear", "Save As...", "Traceback Error"] ("L10n_Parent Menus"), 9:w587) -> ()  [unwired: 2 in, 3 out]
        n264 = event-data() -> ()  [unwired: 2 in, 1 out]
      }
      event "Python Code": Shortcut Menu Activation? {
        n265 = event-data() -> ("MenuRef"=w594:refnum<k9>)  [unwired: 1 in]
        n266 = Delete Menu Items(9:w594) -> (0:w597:errorcluster, 3:w596:refnum<k9>)  [unwired: 3 in]
        n267 = Insert Menu Items(6:w597, 7:string[] ["SPACES", "RUN", "SAVEAS_CODE", "IMPORT_CODE"], 8:string[] ["Check Spaces", "Run in REPL", "Save As...", "Import at end..."] ("L10n_Parent Menus"), 9:w596) -> ()  [unwired: 2 in, 3 out]
        n268 = event-data() -> ()  [unwired: 2 in, 1 out]
      }
      event "Tree", "Console", "Python Code": Shortcut Menu Selection (User); Menu Selection (User) {
        n269 = event-data() -> ("ItemTag"=w606:string)  [unwired: 1 in, 1 out]
        n270 = local read "Tree"() -> (w607:string)
        n271 = case shown="\"IMPORT_CODE\"" w606 {
          tunnel: w608 -> [_ w617 _ w641 w653 w660 w670 w680 w698 _ _ _ _ _ _ _ _ _ w751 _]
          tunnel: w607 -> [_ w612 w627 w639 w643 w658 w662 w677 w692 w717 _ _ _ _ _ _ _ _ _ _]
          tunnel: w605 -> [_ _ _ _ _ _ _ _ _ _ _ w726 _ _ _ _ _ _ _ _]
          tunnel: w604 -> [w609 w611 w626 w638 w642 w657 w661 w679 w691 w706 w718 _ w728 w731 w733 w741 w744 w746 w760 w763]
          tunnel: w603 -> [_ _ _ _ _ _ _ _ _ _ _ w725 _ _ _ _ _ _ _ _]
          tunnel: w602 -> [_ _ _ _ _ _ _ _ _ _ _ _ _ w732 _ _ _ _ _ _]
          tunnel: [w609 w611 w626 w638 w642 w657 w661 w679 w691 w706 w718 "" w728 w731 w733 w741 w744 w745 w760 w763] -> w601
          frame Default {
          }
          frame "NEW" {
            n272 = String To Path(string=w612) -> (path=w616:path)
            n273 = Strip Path(path=w616) -> (stripped path=w615:path)  [unwired: 1 out]
            n274 = call "File Dialog5"("start path"=w615, "default name"="untitled.py") -> ("selected path"=w613:path, "error out"=w614:errorcluster)  [unwired: 10 in, 2 out]
            n275 = case shown="No Error" w614 {
              tunnel: w616 -> [_ _]
              tunnel: w613 -> [w624 _]
              tunnel: w617 -> [w622 _]
              tunnel: [w618 _] -> _
              frame No Error {
                n276 = control-ref of="Tree"() -> (w623:refnum<vi>)
                n277 = call "CheckForExtension.vi"("selected path"=w624) -> ("dup file"=w621:path)  [unwired: 10 in]
                n278 = Write to Text File(file (use dialog)=w621, text="#Enter code") -> (error out=w620:errorcluster)  [unwired: 2 in, 2 out]
                n279 = call "InitializeTree.vi"("Selected File"=w621, "error in (no error)"=w620, "Panel"=w622, "TreeControl in"=w623) -> ("error out"=w618:errorcluster)  [unwired: 6 in, 1 out]
              }
              frame Error {
              }
            }
          }
          frame "OPEN" {
            n280 = String To Path(string=w627) -> (path=w629:path)
            n281 = call <vilib>:"Get File Extension.vi"("file"=w629) -> ("lowercase file extension"=w628:string)  [unwired: 6 in, 4 out]
            n282 = case shown="\"py\"" w628 {
              tunnel: [w635 w637] -> w625
              tunnel: w629 -> [w635 w636]
              frame Default {
              }
              frame "py" {
                n283 = Strip Path(path=w636) -> (stripped path=w637:path)  [unwired: 1 out]
              }
            }
            n284 = disable-structure shown="TARGET_TYPE==Windows" {
              disable-tunnel: w625 -> [w631 w632]
              frame condition #0 {
                n285 = call <vilib>:"Path to URL.vi"("path"=w631) -> ("url"=w630:string)
                n286 = call-poly <vilib>:"Open URL in Default Browser.vi"("URL"=w630) -> ()  [unwired: 5 in, 2 out]
              }
              frame condition #1 (active) {
                n287 = Format Into String(format string="cmd /c explorer.exe \"%s\"", w632) -> (resulting string=w634:string)  [unwired: 2 in, 1 out]
                n288 = call <vilib>:"System Exec.vi"("command line"=w634) -> ()  [unwired: 7 in, 4 out]
              }
            }
          }
          frame "RENAME" {
            n289 = control-ref of="Tree"() -> (w640:refnum<vi>)
            n290 = call "Tree_Rename.vi"("Tree in"=w639, "Panel"=w641, "TreeControl in"=w640) -> ()  [unwired: 9 in]
          }
          frame "DUPLICATE" {
            n291 = String To Path(string=w643) -> (path=w655:path)
            n292 = Strip Path(path=w655) -> (stripped path=w654:path, name=w649:string)
            n293 = Search/Split String(string=w649, search string/char (-)=".py") -> (substring before match=w647:string, match + rest of string=w646:string)  [unwired: 1 in, 1 out]
            n294 = Concatenate Strings(w647, "(1)" ("search string/char (-)"), w646) -> (w645:string)
            n295 = Build Path(base path=w654, name or relative path=w645) -> (appended path=w650:path)
            n296 = control-ref of="Tree"() -> (w652:refnum<vi>)
            n297 = Copy(10:w650, 11:w655) -> (0:w651:errorcluster)  [unwired: 3 in, 2 out]
            n298 = call "InitializeTree.vi"("Selected File"=w650, "error in (no error)"=w651, "Panel"=w653, "TreeControl in"=w652) -> ()  [unwired: 6 in, 2 out]
          }
          frame "RELOAD" {
            n299 = String To Path(string=w658) -> (path=w656:path)
            n300 = control-ref of="Tree"() -> (w659:refnum<vi>)
            n301 = call "InitializeTree.vi"("Selected File"=w656, "Panel"=w660, "TreeControl in"=w659) -> ()  [unwired: 7 in, 2 out]
          }
          frame "DELETE_TREE" {
            n302 = String To Path(string=w662) -> (path=w668:path)
            n303 = Strip Path(path=w668) -> (name=w667:string)  [unwired: 1 out]
            n304 = Format Into String(format string="Are you sure you want to delete the file:  %s?", w667) -> (resulting string=w666:string)  [unwired: 2 in, 1 out]
            n305 = Two Button Dialog(message=w666, 1:"Delete" ("T button name (\"OK\")"), 2:"Cancel" ("T button name (\"OK\")")) -> (T button?=w669:bool)
            n306 = case shown="False" w669 {
              tunnel: w668 -> [w674 _]
              tunnel: w670 -> [w671 _]
              frame False {
                n307 = Delete(path (use dialog)=w674) -> (error out=w672:errorcluster)  [unwired: 4 in, 2 out]
                n308 = control-ref of="Tree"() -> (w673:refnum<vi>)
                n309 = call "InitializeTree.vi"("error in (no error)"=w672, "Panel"=w671, "TreeControl in"=w673) -> ()  [unwired: 7 in, 2 out]
              }
              frame True {
              }
            }
          }
          frame "NEW_TREE" {
            n310 = String To Path(string=w677) -> (path=w676:path)
            n311 = call "File Dialog7"("start path"=w676) -> ("selected path"=w678:path, "error out"=w675:errorcluster)  [unwired: 11 in, 2 out]
            n312 = case shown="No Error" w675 {
              tunnel: w680 -> [w684 _]
              tunnel: w678 -> [w682 _]
              frame No Error {
                n313 = call "CheckForExtension.vi"("selected path"=w682) -> ("dup file"=w681:path)  [unwired: 10 in]
                n314 = call <vilib>:"Check if File or Folder Exists.vi"("path"=w682) -> ("file or folder exists?"=w683:bool)  [unwired: 8 in, 2 out]
                n315 = case shown="False" w683 {
                  tunnel: w684 -> [w688 _]
                  tunnel: w681 -> [w687 _]
                  frame False {
                    n316 = call <vilib>:"Create File and Containing Folders.vi"("file path"=w687) -> ("refnum out"=w686:refnum<file>)  [unwired: 9 in, 1 out]
                    n317 = Write to Text File(file (use dialog)=w686, text="#Enter code\n\n") -> ()  [unwired: 2 in, 3 out]
                    n318 = control-ref of="Tree"() -> (w689:refnum<vi>)
                    n319 = call "InitializeTree.vi"("Selected File"=w687, "Panel"=w688, "TreeControl in"=w689) -> ()  [unwired: 7 in, 2 out]
                  }
                  frame True {
                    n320 = One Button Dialog(message="File already exists") -> ()  [unwired: 1 in, 1 out]
                  }
                }
              }
              frame Error {
              }
            }
          }
          frame "SAVEAS_TREE" {
            n321 = String To Path(string=w692) -> (path=w696:path)
            n322 = Strip Path(path=w696) -> (stripped path=w695:path, name=w697:string)
            n323 = call "File Dialog4"("start path"=w695, "default name"=w697) -> ("selected path"=w693:path, "error out"=w694:errorcluster)  [unwired: 10 in, 2 out]
            n324 = case shown="No Error" w694 {
              tunnel: w696 -> [_ _]
              tunnel: w693 -> [w705 _]
              tunnel: w698 -> [w703 _]
              tunnel: [w699 _] -> _
              frame No Error {
                n325 = control-ref of="Tree"() -> (w704:refnum<vi>)
                n326 = local read "Python Code"() -> (w702:string)
                n327 = call "CheckForExtension.vi"("selected path"=w705) -> ("dup file"=w701:path)  [unwired: 10 in]
                n328 = Write to Text File(file (use dialog)=w701, text=w702) -> (error out=w700:errorcluster)  [unwired: 2 in, 2 out]
                n329 = call "InitializeTree.vi"("Selected File"=w701, "error in (no error)"=w700, "Panel"=w703, "TreeControl in"=w704) -> ("error out"=w699:errorcluster)  [unwired: 6 in, 1 out]
              }
              frame Error {
              }
            }
          }
          frame "WINDOW" {
            w709 = 128  # call and forget
            n330 = String To Path(string=w717) -> (path=w708:path)
            n331 = vi-ref "MainWindow.vi"() -> (w713:refnum<vi>)
            n332 = property class="VI"(reference=w713) -> ("Name"=w712:string)  [unwired: 1 in, 2 out]
            n333 = Open VI Reference(type specifier VI Refnum (for type only)=refnum<vi> refnum, vi path=w712, options=w709) -> (vi reference=w711:refnum<vi>, error out=w716:errorcluster)  [unwired: 3 in]
            n334 = call-by-ref "Start Asynchronous Call"(reference=w711, error in=w716, "Path"=w708) -> (reference out=w715:refnum<vi>, error out=w714:errorcluster)  [unwired: 11 in]
            n335 = property on="Tree" class="Tree (strict)"("Val(Sgnl)"="" ("Value (Signaling)")) -> ()  [unwired: 2 in, 2 out]
            n336 = Close Reference(reference=w715, error in (no error)=w714) -> ()  [unwired: 1 out]
          }
          frame "SAVEAS" {
            n337 = call "File Dialog"("default name"="log.txt") -> ("selected path"=w720:path, "error out"=w721:errorcluster)  [unwired: 11 in, 2 out]
            n338 = case shown="No Error" w721 {
              tunnel: w720 -> [w722 _]
              frame No Error {
                n339 = local read "Console"() -> (w723:string)
                n340 = Write to Text File(file (use dialog)=w722, text=w723) -> ()  [unwired: 2 in, 3 out]
              }
              frame Error {
              }
            }
          }
          frame "CTRLC" {
            n341 = call "Comm_Write.vi"("error in (no error)"=w726, "Text to write"="\u0003\r\n\r\n" ("function name"), "Python"=w725) -> ()  [unwired: 7 in, 2 out]
          }
          frame "CLEAR" {
            n342 = local write "Console"("") -> ()
            n343 = local write "Buffer"(0) -> ()
          }
          frame "ERROR" {
            n344 = call "ErrorWindow.vi"("Console in"=w732) -> ()  [unwired: 10 in]
          }
          frame "SAVEAS_CODE" {
            n345 = local read "Path"() -> (w736:path)
            n346 = Strip Path(path=w736) -> (stripped path=w735:path, name=w734:string)
            n347 = call "File Dialog2"("start path"=w735, "default name"=w734) -> ("selected path"=w737:path, "error out"=w738:errorcluster)  [unwired: 10 in, 2 out]
            n348 = case shown="No Error" w738 {
              tunnel: w737 -> [w739 _]
              frame No Error {
                n349 = local read "Python Code"() -> (w740:string)
                n350 = Write to Text File(file (use dialog)=w739, text=w740) -> ()  [unwired: 2 in, 3 out]
              }
              frame Error {
              }
            }
          }
          frame "SPACES" {
            n351 = property on="Python Code" class="Str"() -> ("Value"=w742:string)  [unwired: 2 in, 2 out]
            n352 = call "CleanUp.vi"("Python Code"=w742) -> ("spreadsheet string"=w743:string)  [unwired: 10 in]
            n353 = property on="Python Code" class="Str"("Val(Sgnl)"=w743) -> ()  [unwired: 2 in, 2 out]
          }
          frame "SEARCH" {
          }
          frame "RUN" {
            n354 = local read "Python Code"() -> (w747:string)
            n355 = local read "Processor"() -> (w748:u16)
            n356 = call "LineByLine.vi"("Processor"=w748, "Python Code"=w747) -> ("result string"=w749:string)  [unwired: 9 in]
            n357 = Concatenate Strings(w746, w749) -> (w745:string)
          }
          frame "FIND" {
            w752 = 128  # call and forget
            n358 = vi-ref "FindnReplace.vi"() -> (w757:refnum<vi>)
            n359 = property class="VI"(reference=w757) -> ("Name"=w758:string)  [unwired: 1 in, 2 out]
            n360 = Open VI Reference(type specifier VI Refnum (for type only)=refnum<vi> refnum, vi path=w758, options=w752) -> (vi reference=w759:refnum<vi>, error out=w754:errorcluster)  [unwired: 3 in]
            n361 = control-ref of="Python Code"() -> (w750:refnum<vi>)
            n362 = call-by-ref "Start Asynchronous Call"(reference=w759, error in=w754, "Front Panel"=w751, "Python Code"=w750) -> (reference out=w755:refnum<vi>, error out=w756:errorcluster)  [unwired: 10 in]
            n363 = Close Reference(reference=w755, error in (no error)=w756) -> ()  [unwired: 1 out]
          }
          frame "IMPORT_CODE" {
            n364 = call "File Dialog6"() -> ("selected path"=w761:path, "cancelled"=w762:bool)  [unwired: 12 in, 2 out]
            n365 = case shown="False" w762 {
              tunnel: w761 -> [w767 _]
              frame False {
                n366 = local read "Python Code"() -> (w766:string)
                n367 = Read from Text File(file (use dialog)=w767) -> (text=w765:string)  [unwired: 3 in, 3 out]
                n368 = Concatenate Strings(w766, w765) -> (w764:string)
                n369 = local write "Python Code"(w764) -> ()
              }
              frame True {
              }
            }
          }
        }
      }
    }
    "Script" <- w68
    "error IO" <- w62
    n370 = Unbundle(w62) -> ("status"=w61:bool)  [unwired: 2 out]
    n371 = Not(x=w61) -> (.not. x?=→"live":bool)
  }
  n372 = property on="Line #" class="Str"() -> ("Top"=w24:i32, "Left"=w22:i32, "Height"=w25:u32, "Width"=w26:u32)  [unwired: 2 in, 2 out]
  n373 = Add(x=w22, y=w27) -> (x+y=w23:i32)
  n374 = Subtract(x=w26, y=w27) -> (x-y=w28:u32)
  n375 = property on="Python Code" class="Str"("Top"=w24, "Left"=w23, "Height"=w25, "Width"=w28) -> ()  [unwired: 2 in, 2 out]
  n376 = disable-structure shown="Enabled" {
    frame Disabled {
      n377 = control-ref of="This VI"() -> (w768:refnum<vi>)
      n378 = property class="VI"(reference=w768, "BDWin.Open"=TRUE ("Block Diagram Window:Open")) -> ()  [unwired: 1 in, 2 out]
    }
    frame Enabled {
    }
  }
  n379 = disable-structure shown="Disabled" {
    frame Disabled {
      n380 = call "MainWindow.vi"() -> ()  [unwired: 12 in]
      n381 = call "Examples.vi"() -> ()  [unwired: 12 in]
      n382 = call "ErrorWindow.vi"() -> ()  [unwired: 11 in]
      n383 = call "SimplePyScriptTests.vi"() -> ()  [unwired: 12 in]
      n384 = call "Demo.vi"() -> ()  [unwired: 12 in]
      n385 = call "MQTT_Client.vi"() -> ()  [unwired: 12 in]
      n386 = call "OpenMV.vi"() -> ()  [unwired: 12 in]
      n387 = call "Image.vi"() -> ()  [unwired: 12 in]
      n388 = call "Spatial Toolbox.vi"() -> ()  [unwired: 12 in]
      n389 = call "OnshapeTwin.vi"() -> ()  [unwired: 12 in]
      n390 = call "Twin.vi"() -> ()  [unwired: 12 in]
      n391 = call "Scope.vi"() -> ()  [unwired: 12 in]
      n392 = call "Arm.vi"() -> ()  [unwired: 12 in]
      n393 = call "Pinouts.vi"() -> ()  [unwired: 12 in]
      n394 = call "Tektronix.vi"() -> ()  [unwired: 12 in]
      n395 = call "Motors.vi"() -> ()  [unwired: 12 in]
      n396 = call "ROS2.vi"() -> ()  [unwired: 12 in]
      n397 = call "Backpack.vi"() -> ()  [unwired: 12 in]
    }
    frame Enabled {
    }
  }
  n398 = disable-structure shown="Disabled" {
    frame Disabled {
      n399 = call "serialPorts.vi"() -> ()  [unwired: 8 in, 4 out]
      n400 = call "serialInit.vi"() -> ("error out"=w772:errorcluster, "port name"=w771:string)  [unwired: 9 in, 1 out]
      n401 = call "serialWrite.vi"("error in (no error)"=w772, "text"=w771) -> ("error out"=w770:errorcluster)  [unwired: 7 in, 2 out]
      n402 = call "serialRead.vi"("error in (no error)"=w770) -> ()  [unwired: 8 in, 3 out]
      n403 = call "serialClose.vi"() -> ()  [unwired: 10 in, 2 out]
    }
    frame Enabled {
    }
  }
  n404 = Not Equal?(x=w10, y=w9) -> (x != y?=w8:T11)
  n405 = Unbundle By Name(w8) -> ()  [unwired: 1 out]
  n406 = call "Comm_Close.vi"("error in (no error)"=w10, "Show Err?"=FALSE, "Python in"=w13) -> ("error out"=w12:errorcluster)  [unwired: 7 in, 1 out]
  n407 = flat-sequence {
    tunnel: w12 -> [_]
    frame #0 {
    }
  }
